vi "Stepper.vi"(8 "error in":errorcluster, 9 "Axis Queue":refnum<queue>, 10 "UI Queue":refnum<queue>) -> (0 "error out":errorcluster)   [LabVIEW 2016, in "SMD-7615.lvlib"]
uses:
  SMD-7615.lvlib
  support/Message Queue/Message Cluster.ctl
  CTL/Stepper Drive Config.ctl
  CTL/SV General.ctl
  CTL/SV Inputs.ctl
  CTL/SV Outputs.ctl
  CTL/Motion IO.ctl
  CTL/Digital Lines (Read).ctl
  CTL/Status.ctl
  CTL/Encoder.ctl
  CTL/Position.ctl
  <vilib>/Motion/PropertyNodes/nimc.createStraightLineMoveInstance.axis.vi
  <vilib>/GPower/Error/Library/Append/AppendSingle.vi
  support/Message Queue/Enqueue Message (Single).vi
  <vilib>/Motion/PropertyNodes/nimc.destroyInterfaceInstance.vi
  <vilib>/ErrorRing/Error Ring.xnode
  support/Message Queue/Message Queue.lvlib
  <resource>/objmgr/nimotion.rc
  <resource>/objmgr/nimcca.rc
  <vilib>/GPower/Error/GPError.lvlib
  LUL-All/LUL-Syslog/LUL-SysLog.lvlib
panel:
  out "Timeout Counter":i32
  out "Stall detected (Software)":bool
  out "Moving ? (Software)":bool
  out "Position":T1
  out "Encoder":T2
  out "Status":T3
  in  "Stop Button":bool
  out "Axis Name":string
  out "Digital Lines (Read)":T4
  out "Motion I/O":T5
  out "dt DAQ Loop (ms)":u32
  out "Axis Config Constant":T6
  out "Last Received SV Update":timestamp
  out "Exit ?":bool
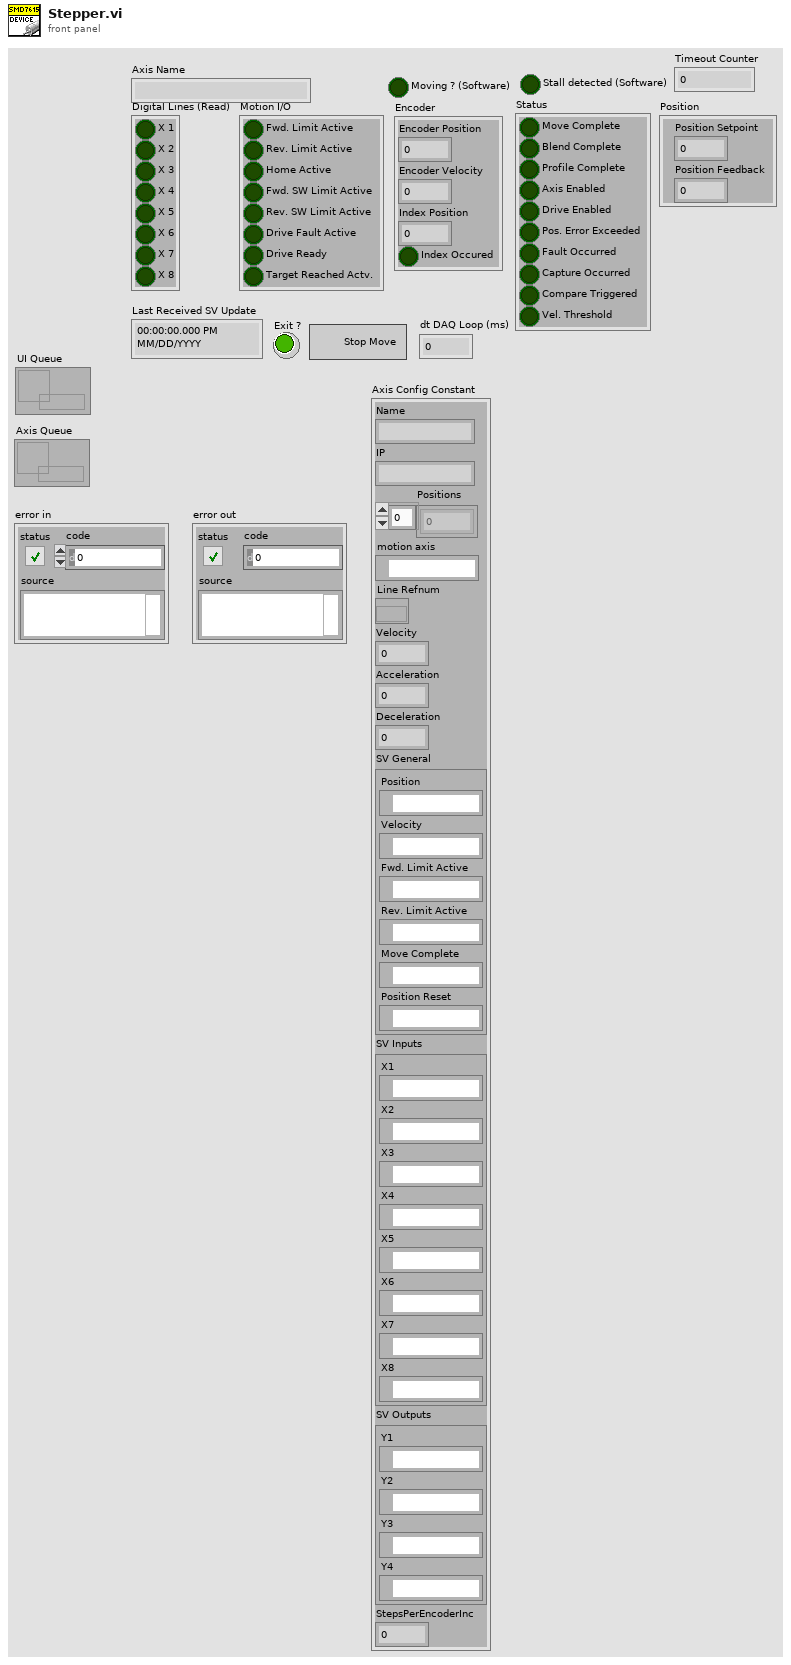
[diagram p1: front panel]
types:
  T1 = typedef "SMD-7615.lvlib/Position.ctl" = cluster{"Position Setpoint":dbl, "Position Feedback":dbl}
  T2 = typedef "SMD-7615.lvlib/Encoder.ctl" = cluster{"Encoder Position":dbl, "Encoder Velocity":dbl, "Index Position":dbl, "Index Occured":bool}
  T3 = typedef "SMD-7615.lvlib/Status.ctl" = cluster{"Move Complete":bool, "Blend Complete":bool, "Profile Complete":bool, "Axis Enabled":bool, "Drive Enabled":bool, "Pos. Error Exceeded":bool, "Fault Occurred":bool, "Capture Occurred":bool, "Compare Triggered":bool, "Vel. Threshold":bool}
  T4 = typedef "SMD-7615.lvlib/Digital Lines (Read).ctl" = cluster{"X 1":bool, "X 2":bool, "X 3":bool, "X 4":bool, "X 5":bool, "X 6":bool, "X 7":bool, "X 8":bool}
  T5 = typedef "SMD-7615.lvlib/Motion IO.ctl" = cluster{"Fwd. Limit Active":bool, "Rev. Limit Active":bool, "Home Active":bool, "Fwd. SW Limit Active":bool, "Rev. SW Limit Active":bool, "Drive Fault Active":bool, "Drive Ready":bool, "Target Reached Actv.":bool}
  T6 = typedef "SMD-7615.lvlib/Stepper Drive Config.ctl" = cluster{"Name":string, "IP":string, "Positions":dbl[], "motion axis ":refnum<k21>, "Line Refnum":refnum<k20>, "Velocity":dbl, "Acceleration":dbl, "Deceleration":dbl, "SV General":T7, "SV Inputs":T8, "SV Outputs":T9, "StepsPerEncoderInc":i32}
  T7 = typedef "SMD-7615.lvlib/SV General.ctl" = cluster{"Position":refnum<k21>, "Velocity":refnum<k21>, "Fwd. Limit Active":refnum<k21>, "Rev. Limit Active":refnum<k21>, "Move Complete":refnum<k21>, "Position Reset":refnum<k21>}
  T8 = typedef "SMD-7615.lvlib/SV Inputs.ctl" = cluster{"X1":refnum<k21>, "X2":refnum<k21>, "X3":refnum<k21>, "X4":refnum<k21>, "X5":refnum<k21>, "X6":refnum<k21>, "X7":refnum<k21>, "X8":refnum<k21>}
  T9 = typedef "SMD-7615.lvlib/SV Outputs.ctl" = cluster{"Y1":refnum<k21>, "Y2":refnum<k21>, "Y3":refnum<k21>, "Y4":refnum<k21>}
  T10 = typedef "Semaphore RefNum" = refnum<k1>
  T11 = typedef "SMD-7615.lvlib/Axis Data.ctl" = cluster{"Motion I/O":T5, "Digital Lines (Read)":T4, "Status":T3, "Encoder":T2, "Position":T1, "Moving ? (Software)":bool, "Stall detected (Software)":bool}
  T12 = enum32{"Invalid", "Standard", "Closed", "Hidden", "Minimized", "Maximized"}
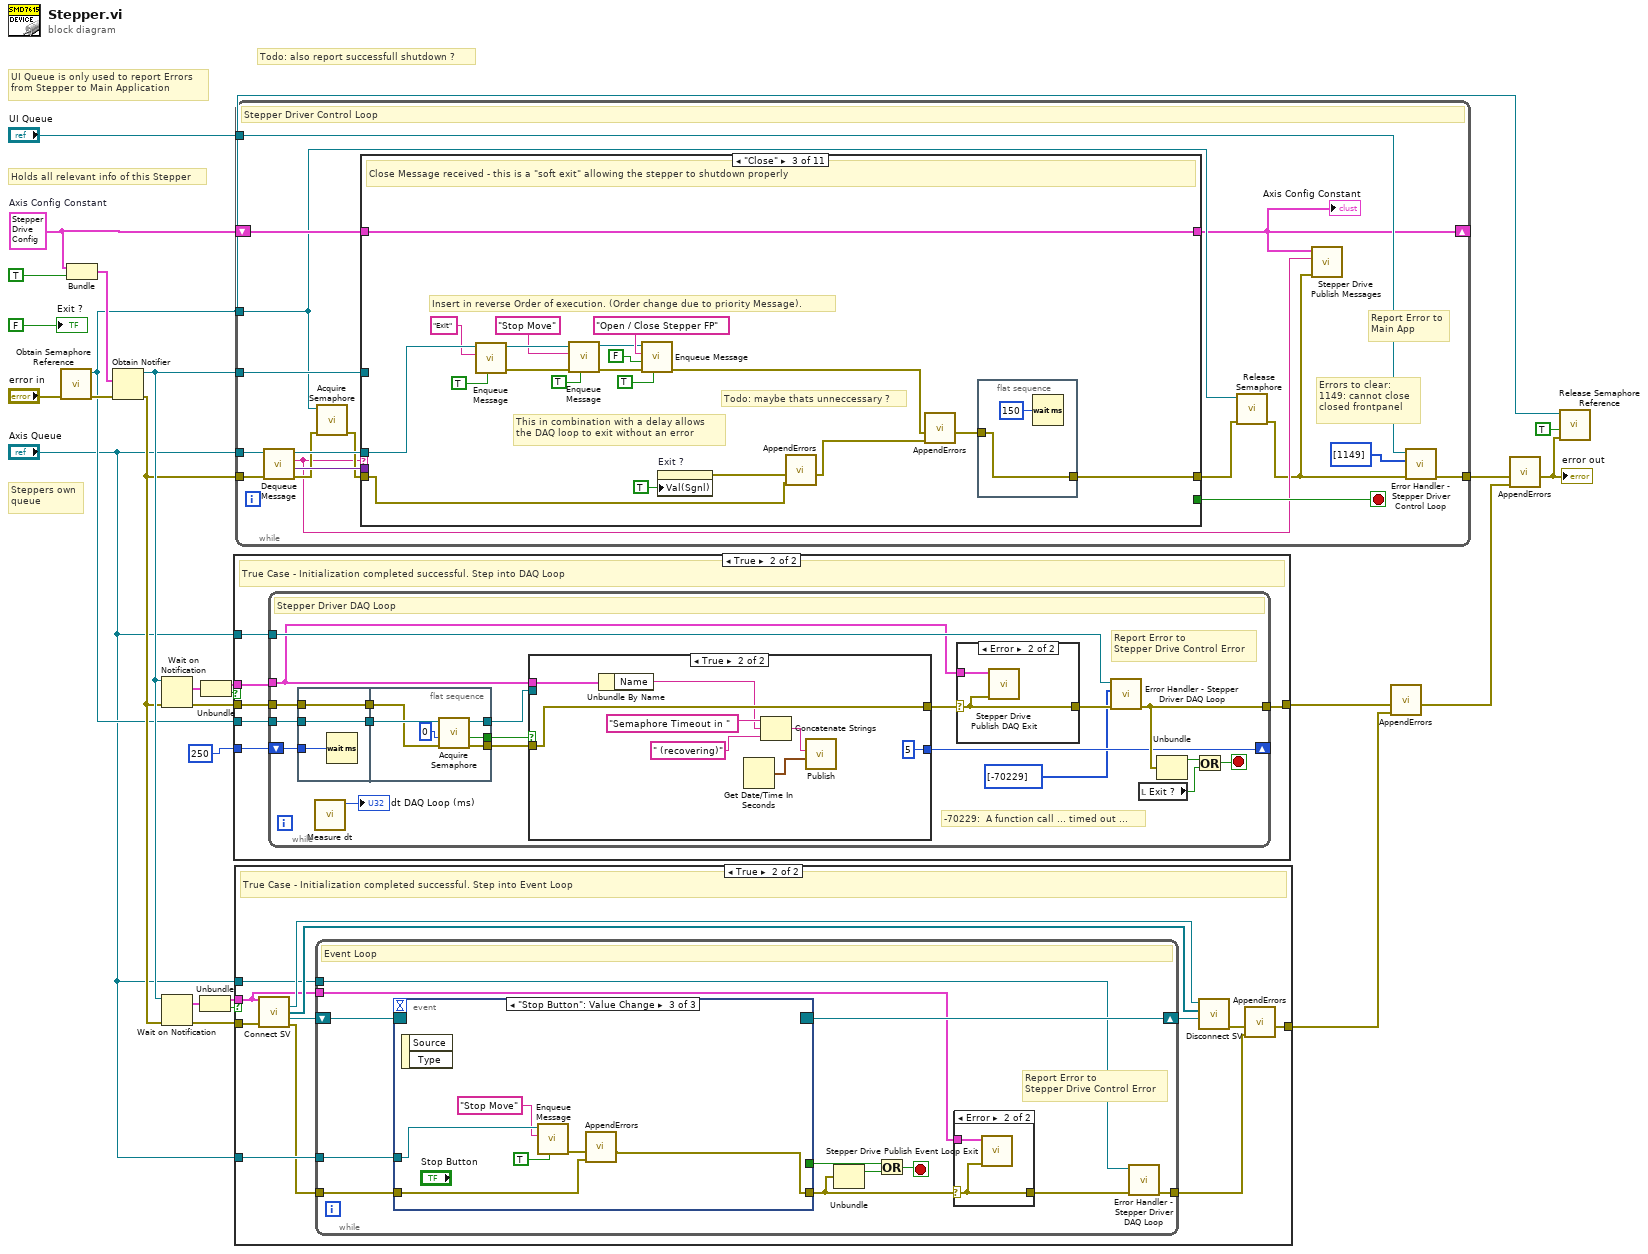
[diagram p0: block diagram]
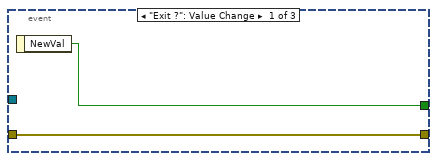
[diagram p4: hidden frame]
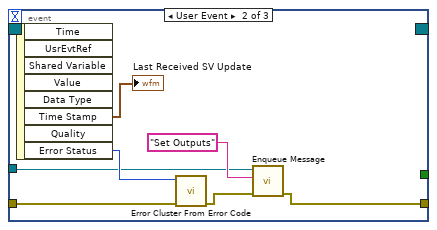
[diagram p5: hidden frame]
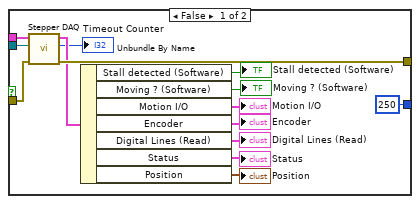
[diagram p8: hidden frame]
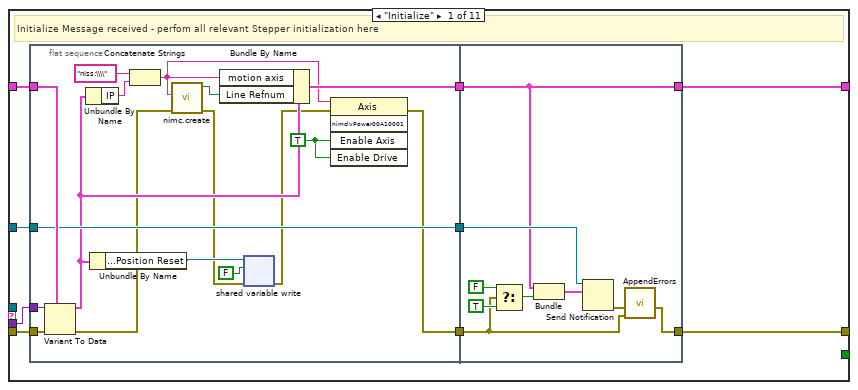
[diagram p9: hidden frame]
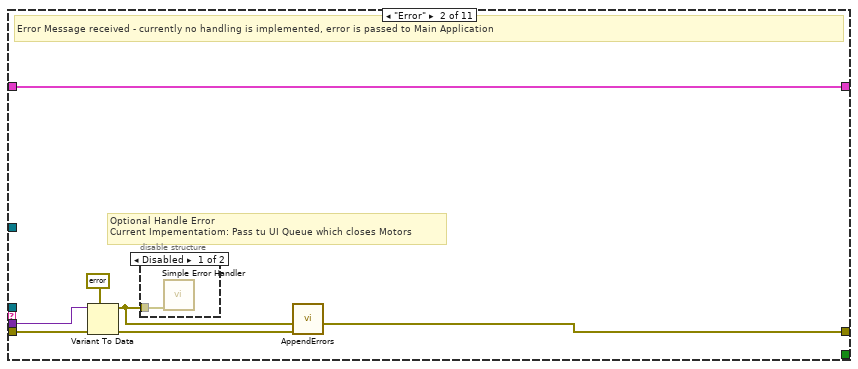
[diagram p10: hidden frame]
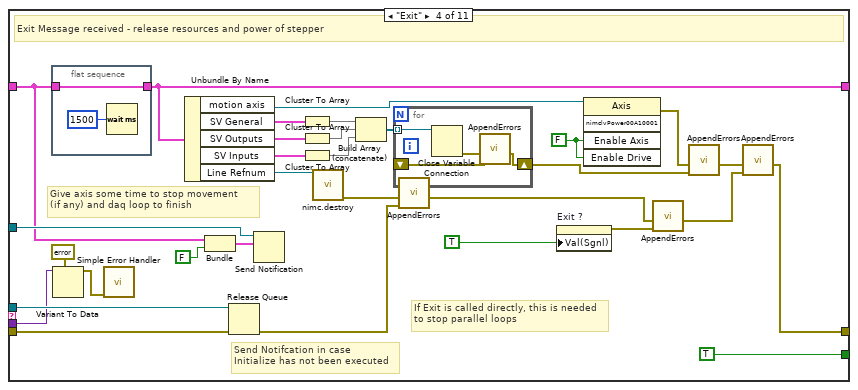
[diagram p12: hidden frame]
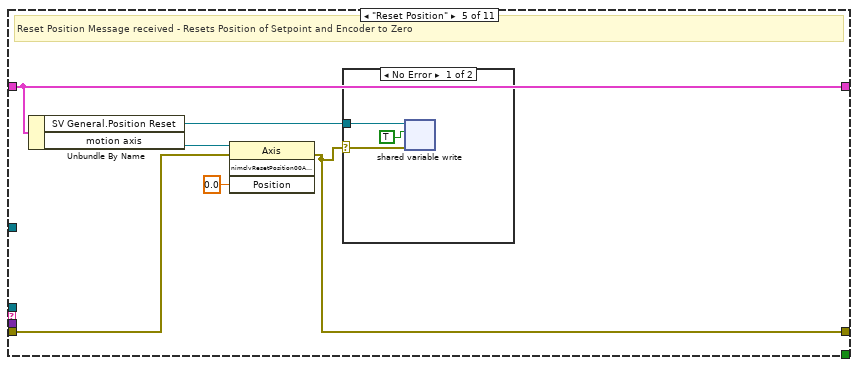
[diagram p13: hidden frame]
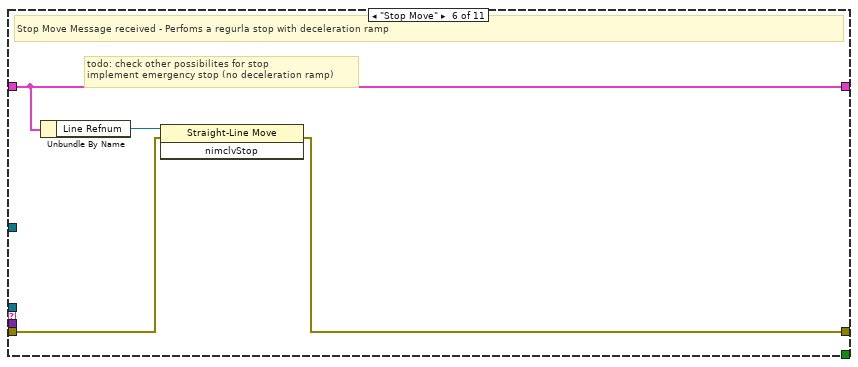
[diagram p15: hidden frame]
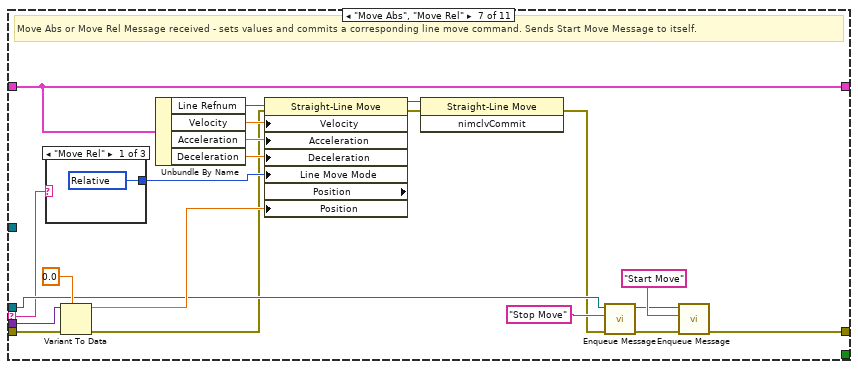
[diagram p16: hidden frame]
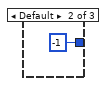
[diagram p17: hidden frame]
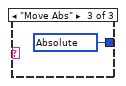
[diagram p18: hidden frame]
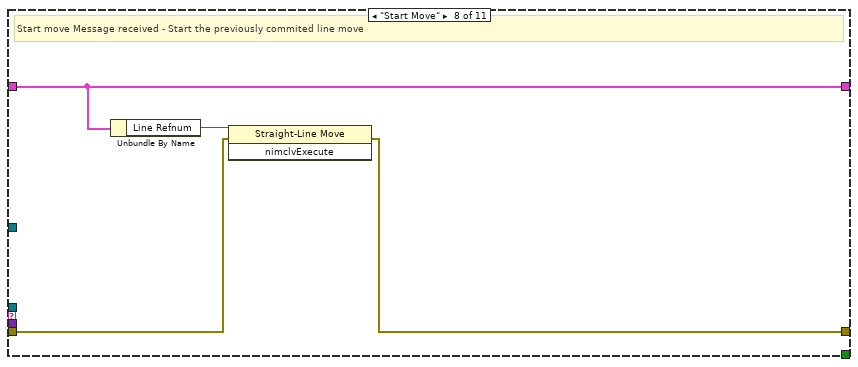
[diagram p19: hidden frame]
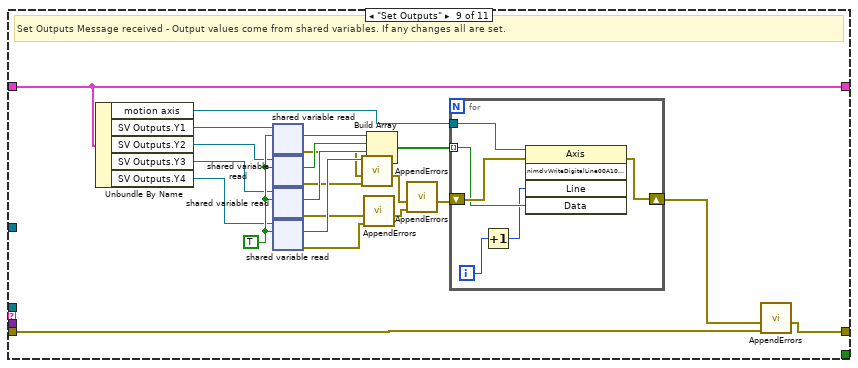
[diagram p20: hidden frame]
diagram:
  w11 = T6 {"Name"="", "IP"="", "Positions"=[], "motion axis "="", "Line Refnum"=refnum, "Velocity"=0.0, "Acceleration"=0.0, "Deceleration"=0.0, "SV General"={"Position"="", "Velocity"="", "Fwd. Limit Active"="", "Rev. Limit Active"="", "Move Complete"="", "Position Reset"=""}, "SV Inputs"={"X1"="", "X2"="", "X3"="", "X4"="", "X5"="", "X6"="", "X7"="", "X8"=""}, "SV Outputs"={"Y1"="", "Y2"="", "Y3"="", "Y4"=""}, "StepsPerEncoderInc"=0}  # Axis Config Constant
  # "Steppers own\nqueue"
  # "Holds all relevant info of this Stepper"
  # "Todo: also report successfull shutdown ?"
  # "UI Queue is only used to report Errors\nfrom Stepper to Main Application"
  n1 = call <vilib>:"Obtain Semaphore Reference.vi"("error in (no error)"="error in") -> ("error out"=w9:errorcluster, "semaphore"=w7:T10)  [unwired: 4 in, 1 out]
  n2 = Bundle("Axis Config Constant"=w11, TRUE) -> (w22:cluster{"Axis Config Constant":T6, bool})  [unwired: 1 in]
  n3 = Obtain Notifier(notification data type=w22, error in (no error)=w9) -> (notifier out=w23:refnum<notifier>, error out=w10:errorcluster)  [unwired: 2 in, 1 out]
  n4 = Wait on Notification(notifier=w23, error in (no error)=w10) -> (notification=w20:cluster{"Axis Config Constant":T6, bool}, error out=w25:errorcluster)  [unwired: 2 in, 2 out]
  n5 = Wait on Notification(notifier=w23, error in (no error)=w10) -> (notification=w17:cluster{"Axis Config Constant":T6, bool}, error out=w24:errorcluster)  [unwired: 2 in, 2 out]
  n6 = Unbundle(w17) -> ("Axis Config Constant"=w15:T6, w16:bool)
  n7 = Unbundle(w20) -> ("Axis Config Constant"=w18:T6, w19:bool)
  n8 = case shown="True" w19 {
    tunnel: [w27 w33] -> w5
    tunnel: "Axis Queue" -> [_ w32]
    tunnel: w25 -> [w27 w31]
    tunnel: w18 -> [_ w30]
    tunnel: w7 -> [_ w29]
    tunnel: u32 250 ("millisecond multiple") -> [_ w28]
    frame False {
      # "False Case - Initialization not successful. Skip DAQ Loop"
    }
    frame True {
      # "True Case - Initialization completed successful. Step into DAQ Loop"
      n9 = while {
        tunnel: w31 -> [w40]
        tunnel: [w51] -> w33
        tunnel: w32 -> [w52]
        tunnel: w30 -> [w35]
        tunnel: w29 -> [w43]
        shift-right: [w38] -> _
        shift-left: w28 -> [w39]
        stop <- w48 stop-if-true
        # "-70229:  A function call ... timed out ..."
        # "Report Error to\nStepper Drive Control Error"
        # "Stepper Driver DAQ Loop"
        n10 = flat-sequence {
          tunnel: w43 -> [w58]
          tunnel: [w58] -> w42
          tunnel: [w57] -> w41
          tunnel: w40 -> [w57]
          tunnel: w39 -> [w56]
          tunnel: [w63] -> w46
          tunnel: [w62] -> w45
          tunnel: [w61] -> w44
          tunnel: w42 -> [w60]
          tunnel: w41 -> [w59]
          frame #0 {
            n11 = Wait (ms)(milliseconds to wait=w56) -> ()  [unwired: 1 out]
          }
          frame #1 {
            n12 = call <vilib>:"Acquire Semaphore.vi"("error in (no error)"=w59, "ms timeout (-1)"=0, "semaphore"=w60) -> ("error out"=w61:errorcluster, "timed out"=w63:bool, "semaphore out"=w62:T10)  [unwired: 2 in]
          }
        }
        n13 = call "Measure dt.vi"() -> ("dt"=→"dt DAQ Loop (ms)":u32)  [unwired: 11 in]
        n14 = case shown="True" w46 {
          tunnel: [w78 w85] -> w37
          tunnel: w35 -> [w68 w83]
          tunnel: w45 -> [w67 _]
          tunnel: w44 -> [w66 w85]
          tunnel: [u32 250 ("millisecond multiple") u32 5 ("millisecond multiple")] -> w38
          frame False {
            n15 = call "Stepper DAQ.vi"("error in"=w66, "semaphore"=w67, "BIBA 2017 Config"=w68) -> ("error out"=w78:errorcluster, "Timeout Counter"=→"Timeout Counter":i32, "Axis Data"=w77:T11)  [unwired: 6 in]
            n16 = Unbundle By Name(w77) -> ("Stall detected (Software)"=→"Stall detected (Software)":bool, "Moving ? (Software)"=→"Moving ? (Software)":bool, "Motion I/O"=→"Motion I/O":T5, "Encoder"=→"Encoder":T2, "Digital Lines (Read)"=→"Digital Lines (Read)":T4, "Status"=→"Status":T3, "Position"=→"Position":T1)
          }
          frame True {
            n17 = Unbundle By Name(w83) -> ("Name"=w81:string)
            n18 = Get Date/Time In Seconds() -> (seconds since 1Jan1904=w84:timestamp)
            n19 = Concatenate Strings("Semaphore Timeout in " ("Message"), w81, " (recovering)" ("string")) -> (w80:string)
            n20 = call "Publish.vi"("current time"=w84, "Message"=w80) -> ()  [unwired: 9 in, 1 out]
          }
        }
        n21 = case shown="Error" w37 {
          selector: w37 -> [w53 w55]
          tunnel: [w53 w55] -> w36
          tunnel: w35 -> [_ w54]
          frame No Error {
          }
          frame Error {
            n22 = call "Stepper Drive Publish DAQ Exit.vi"("error in (no error)"=w55, "Axis Config Constant"=w54) -> ()  [unwired: 10 in]
          }
        }
        n23 = call "Error Handler - Stepper Driver DAQ Loop.vi"("error in (no error)"=w36, "Ignore Errors (Runtime)"=i32[] [-70229], "Message Queue"=w52) -> ("dup error in"=w51:errorcluster)  [unwired: 7 in, 1 out]
        n24 = local read "Exit ?"() -> (w49:bool)
        n25 = Unbundle(w51) -> ("status"=w50:bool)  [unwired: 2 out]
        n26 = Or(x=w50, y=w49) -> (x .or. y?=w48:bool)
      }
    }
  }
  n27 = case shown="True" w16 {
    tunnel: "Axis Queue" -> [_ w99]
    tunnel: [w87 w91] -> w4
    tunnel: w24 -> [w87 w98]
    tunnel: w15 -> [_ w88]
    tunnel: "Axis Queue" -> [_ w89]
    frame False {
      # "False Case - Initialization not successful. Skip Event Loop"
    }
    frame True {
      # "True Case - Initialization completed successful. Step into Event Loop"
      n28 = call "Connect SV.vi"("Axis Config in"=w88, "Error In"=w98) -> ("shared variable value change notification"=w95:refnum<user-event>, "Shared Variables"=w93:refnum<k21>[], "Event Registration Refnum"=w96:refnum<event-registration>, "Error Out"=w97:errorcluster)  [unwired: 9 in, 1 out]
      n29 = while {
        tunnel: w99 -> [w109]
        tunnel: w97 -> [w111]
        tunnel: [w104] -> w92
        shift-right: [w108] -> w94
        shift-left: w96 -> [w110]
        tunnel: w89 -> [w102]
        tunnel: w88 -> [w101]
        stop <- w106 stop-if-true
        # "Report Error to\nStepper Drive Control Error"
        # "Event Loop"
        n30 = event shown="[2] \"Stop Button\": Value Change" {
          selector: w110 -> [_ _ _]
          dyn-events: [_ _ _] -> w108
          timeout: _ -> [_ _ _]
          tunnel: w111 -> [w116 w121 w125]
          tunnel: [w116 w117 w126] -> w103
          tunnel: w109 -> [_ w119 w128]
          tunnel: [w115 _ _] -> w105
          event "Exit ?": Value Change {
            n31 = event-data() -> ("NewVal"=w115:bool)  [unwired: 1 in]
          }
          event User Event {
            n32 = event-data() -> ("Time Stamp"=→"Last Received SV Update":timestamp, "Error Status"=w120:i32)  [unwired: 1 in, 6 out]
            n33 = call <vilib>:"Error Cluster From Error Code.vi"("error in (no error)"=w121, "error code (0)"=w120) -> ("error out"=w122:errorcluster)  [unwired: 1 in, 6 out]
            n34 = call-poly "Enqueue Message.vi"("error in (no error)"=w122, "Message"="Set Outputs", "Message Queue"=w119) -> ("error out"=w117:errorcluster)  [unwired: 7 in, 1 out]
          }
          event "Stop Button": Value Change {
            n35 = event-data() -> ()  [unwired: 1 in, 2 out]
            n36 = call-poly "Enqueue Message.vi"("Priority Message? (F)"=TRUE, "Message"="Stop Move", "Message Queue"=w128) -> ("error out"=w124:errorcluster)  [unwired: 7 in, 1 out]
            n37 = call-poly <vilib>:"AppendErrors.vi"("Error to append"=w125, "Error in"=w124) -> ("Appended errors out"=w126:errorcluster)  [unwired: 9 in]
          }
        }
        n38 = Unbundle(w103) -> ("status"=w107:bool)  [unwired: 2 out]
        n39 = Or(x=w105, y=w107) -> (x .or. y?=w106:bool)
        n40 = case shown="Error" w103 {
          selector: w103 -> [w112 w113]
          tunnel: w101 -> [_ w114]
          tunnel: [w112 w113] -> w100
          frame No Error {
          }
          frame Error {
            n41 = call "Stepper Drive Publish Event Loop Exit.vi"("error in (no error)"=w113, "Axis Config Constant"=w114) -> ()  [unwired: 10 in]
          }
        }
        n42 = call "Error Handler - Stepper Driver DAQ Loop.vi"("error in (no error)"=w100, "Message Queue"=w102) -> ("dup error in"=w104:errorcluster)  [unwired: 8 in, 1 out]
      }
      n43 = call "Disconnect SV.vi"("Event Registration Refnum"=w94, "Shared Variables"=w93, "User Event in"=w95) -> ("error out"=w90:errorcluster)  [unwired: 8 in]
      n44 = call-poly <vilib>:"AppendErrors.vi"("Error to append"=w92, "Error in"=w90) -> ("Appended errors out"=w91:errorcluster)  [unwired: 9 in]
    }
  }
  n45 = while {
    tunnel: "Axis Queue" -> [w146]
    tunnel: w10 -> [w145]
    tunnel: [w141] -> w13
    shift-right: [w132] -> _
    shift-left: w11 -> [w142]
    tunnel: "UI Queue" -> [w140]
    tunnel: w23 -> [w138]
    tunnel: w7 -> [w133]
    stop <- w143 stop-if-true
    # "Report Error to\nMain App"
    # "Errors to clear:\n1149: cannot close \nclosed frontpanel"
    # "Stepper Driver Control Loop"
    n46 = call "Dequeue Message.vi"("error in (no error)"=w145, "Message Queue"=w146) -> ("error out"=w136:errorcluster, "Message Data"=w144:variant, "Message"=w131:string, "dup Message Queue"=w139:refnum<queue>)  [unwired: 6 in]
    n47 = call <vilib>:"Acquire Semaphore.vi"("error in (no error)"=w136, "semaphore"=w133) -> ("error out"=w135:errorcluster)  [unwired: 3 in, 2 out]
    n48 = case shown="\"Close\"" w131 {
      selector: w131 -> [_ _ _ _ _ _ w266 _ _ _ w339]
      tunnel: w144 -> [w154 w186 _ w238 _ _ w279 _ _ w326 _]
      tunnel: w135 -> [w155 w185 w194 w240 w251 w261 w282 w287 w297 w327 w335]
      tunnel: [w153 w184 w200 w217 w250 w258 w262 w286 w299 w318 w334] -> w134
      tunnel: w139 -> [_ _ w208 w239 _ _ w269 _ _ _ _]
      tunnel: [_ _ _ TRUE _ _ _ _ _ _ _] -> w143
      tunnel: w142 -> [w152 w188 w209 w213 w253 w260 w281 w289 w311 w321 w338]
      tunnel: [w150 w188 w209 w216 w253 w260 w281 w289 w311 w321 w338] -> w132
      tunnel: w138 -> [w147 _ _ w214 _ _ _ _ _ _ _]
      frame "Initialize" {
        # "Initialize Message received - perfom all relevant Stepper initialization here"
        n49 = flat-sequence {
          tunnel: w155 -> [w172]
          tunnel: w154 -> [w171]
          tunnel: w152 -> [w168]
          tunnel: [w163] -> w151
          tunnel: [w165] -> w149
          tunnel: [w166] -> w148
          tunnel: w147 -> [w166]
          tunnel: [w173] -> w153
          tunnel: w151 -> [w174]
          tunnel: [w178] -> w150
          tunnel: w149 -> [w178]
          tunnel: w148 -> [w179]
          frame #0 {
            w162 = TRUE ("Enable Axis")
            n50 = Variant To Data(error in=w172, type=w168, Variant=w171) -> (data=w160:T6, error out=w156:errorcluster)
            n51 = Unbundle By Name(w160) -> ("IP"=w169:string)
            n52 = Unbundle By Name(w160) -> ("SV General.Position Reset"=w159:refnum<k21>)
            n53 = Concatenate Strings("niss:\\\\" ("string"), w169) -> (w164:string)
            n54 = call-poly <vilib>:"nimc.create.vi"("error in"=w156, "axis"=w164) -> ("error out"=w158:errorcluster, "line"=w167:refnum<k20>)  [unwired: 7 in, 1 out]
            n55 = Bundle By Name(cluster=w160, "motion axis"=w164, "Line Refnum"=w167) -> (w165:T6)
            n56 = shared-variable-write(w159, w158, FALSE) -> (w157:errorcluster)  [unwired: 1 out]
            n57 = invoke class="Axis" method="nimclvPower00A10001"(reference=w164, error in=w157, "Enable Axis"=w162, "Enable Drive"=w162) -> (error out=w163:errorcluster)  [unwired: 1 in, 4 out]
          }
          frame #1 {
            n58 = Select(t=FALSE ("Stepper Init Done"), s=w174, f=TRUE) -> (s? t:f=w177:bool)
            n59 = Bundle("Axis Config Constant"=w178, "f"=w177) -> (w176:cluster{"Axis Config Constant":T6, "f":bool})  [unwired: 1 in]
            n60 = Send Notification(notification=w176, notifier=w179) -> (error out=w175:errorcluster)  [unwired: 1 in, 1 out]
            n61 = call-poly <vilib>:"AppendErrors.vi"("Error to append"=w174, "Error in"=w175) -> ("Appended errors out"=w173:errorcluster)  [unwired: 9 in]
          }
        }
      }
      frame "Error" {
        # "Optional Handle Error\nCurrent Impementatiom: Pass tu UI Queue which closes Motors"
        # "Error Message received - currently no handling is implemented, error is passed to Main Application"
        n62 = Variant To Data(error in=w185, type=errorcluster {"status"=FALSE, "code"=0, "source"=""} ("error constant"), Variant=w186) -> (data=w183:errorcluster, error out=w182:errorcluster)
        n63 = disable-structure shown="Disabled" {
          disable-tunnel: w183 -> [w189 _]
          frame Disabled {
            n64 = call <vilib>:"Simple Error Handler.vi"("error in (no error)"=w189) -> ()  [unwired: 4 in, 5 out]
          }
          frame Enabled {
          }
        }
        n65 = call-poly <vilib>:"AppendErrors.vi"("Error to append"=w182, "Error in"=w183) -> ("Appended errors out"=w184:errorcluster)  [unwired: 9 in]
      }
      frame "Close" {
        # "Todo: maybe thats unneccessary ?"
        # "This in combination with a delay allows\nthe DAQ loop to exit without an error"
        # "Insert in reverse Order of execution. (Order change due to priority Message)."
        # "Close Message received - this is a \"soft exit\" allowing the stepper to shutdown properly"
        n66 = call-poly "Enqueue Message.vi"("Priority Message? (F)"=TRUE, "Message"="Exit", "Message Queue"=w208) -> ("error out"=w203:errorcluster, "dup Message Queue"=w204:refnum<queue>)  [unwired: 7 in]
        n67 = call-poly "Enqueue Message.vi"("Priority Message? (F)"=TRUE, "error in (no error)"=w203, "Message"="Stop Move", "Message Queue"=w204) -> ("error out"=w197:errorcluster, "dup Message Queue"=w198:refnum<queue>)  [unwired: 6 in]
        n68 = call-poly "Enqueue Message.vi"("Priority Message? (F)"=TRUE, "error in (no error)"=w197, "Message Data"=FALSE, "Message"="Open / Close Stepper FP", "Message Queue"=w198) -> ("error out"=w192:errorcluster)  [unwired: 5 in, 1 out]
        n69 = property on="Exit ?" class="Bool (strict)"("Val(Sgnl)"=TRUE ("Value (Signaling)")) -> (error out=w195:errorcluster)  [unwired: 2 in, 1 out]
        n70 = call-poly <vilib>:"AppendErrors.vi"("Error to append"=w194, "Error in"=w195) -> ("Appended errors out"=w191:errorcluster)  [unwired: 9 in]
        n71 = call-poly <vilib>:"AppendErrors.vi"("Error to append"=w191, "Error in"=w192) -> ("Appended errors out"=w193:errorcluster)  [unwired: 9 in]
        n72 = flat-sequence {
          tunnel: [w210] -> w200
          tunnel: w193 -> [w210]
          frame #0 {
            n73 = Wait (ms)(milliseconds to wait=u32 150) -> ()  [unwired: 1 out]
          }
        }
      }
      frame "Exit" {
        w228 = FALSE ("Enable Axis")
        # "Send Notifcation in case\nInitialize has not been executed"
        # "Give axis some time to stop movement \n(if any) and daq loop to finish"
        # "If Exit is called directly, this is needed\nto stop parallel loops"
        # "Exit Message received - release resources and power of stepper"
        n74 = flat-sequence {
          tunnel: w213 -> [w243]
          tunnel: [w243] -> w216
          frame #0 {
            n75 = Wait (ms)(milliseconds to wait=u32 1500) -> ()  [unwired: 1 out]
          }
        }
        n76 = Variant To Data(type=errorcluster {"status"=FALSE, "code"=0, "source"=""} ("error constant"), Variant=w238) -> (data=w241:errorcluster)  [unwired: 1 in, 1 out]
        n77 = call <vilib>:"Simple Error Handler.vi"("error in (no error)"=w241) -> ()  [unwired: 4 in, 5 out]
        n78 = Unbundle By Name(w216) -> ("motion axis"=w227:refnum<k21>, "SV General"=w236:T7, "SV Outputs"=w232:T9, "SV Inputs"=w233:T8, "Line Refnum"=w237:refnum<k20>)
        n79 = Bundle("Axis Config Constant"=w213, FALSE) -> (w215:cluster{"Axis Config Constant":T6, bool})  [unwired: 1 in]
        n80 = Release Queue(queue=w239, error in (no error)=w240) -> (error out=w222:errorcluster)  [unwired: 1 in, 2 out]
        n81 = Send Notification(notification=w215, notifier=w214) -> ()  [unwired: 1 in, 2 out]
        n82 = Cluster To Array(cluster=w236) -> (array=w235:refnum<k21>[])
        n83 = Cluster To Array(cluster=w232) -> (array=w231:refnum<k21>[])
        n84 = Cluster To Array(cluster=w233) -> (array=w230:refnum<k21>[])
        n85 = call-poly <vilib>:"nimc.destroy.vi"("motion handle"=w237) -> ("error out"=w223:errorcluster)  [unwired: 10 in]
        n86 = Build Array (concatenate)(w235, w231, w230) -> (w234:refnum<k21>[])
        n87 = for {
          tunnel: w234 -> [w248] mode=indexing
          shift-right: [w246] -> w224
          shift-left: _ -> [w245]
          n88 = Close Variable Connection(11:w248) -> (0:w247:errorcluster)  [unwired: 1 in]
          n89 = call-poly <vilib>:"AppendErrors.vi"("Error to append"=w245, "Error in"=w247) -> ("Appended errors out"=w246:errorcluster)  [unwired: 9 in]
        }
        n90 = call-poly <vilib>:"AppendErrors.vi"("Error to append"=w222, "Error in"=w223) -> ("Appended errors out"=w220:errorcluster)  [unwired: 9 in]
        n91 = property on="Exit ?" class="Bool (strict)"("Val(Sgnl)"=TRUE ("Value (Signaling)")) -> (error out=w221:errorcluster)  [unwired: 2 in, 1 out]
        n92 = invoke class="Axis" method="nimclvPower00A10001"(reference=w227, "Enable Axis"=w228, "Enable Drive"=w228) -> (error out=w225:errorcluster)  [unwired: 2 in, 4 out]
        n93 = call-poly <vilib>:"AppendErrors.vi"("Error to append"=w221, "Error in"=w220) -> ("Appended errors out"=w219:errorcluster)  [unwired: 9 in]
        n94 = call-poly <vilib>:"AppendErrors.vi"("Error to append"=w224, "Error in"=w225) -> ("Appended errors out"=w218:errorcluster)  [unwired: 9 in]
        n95 = call-poly <vilib>:"AppendErrors.vi"("Error to append"=w219, "Error in"=w218) -> ("Appended errors out"=w217:errorcluster)  [unwired: 9 in]
      }
      frame "Reset Position" {
        # "Reset Position Message received - Resets Position of Setpoint and Encoder to Zero"
        n96 = Unbundle By Name(w253) -> ("SV General.Position Reset"=w249:refnum<k21>, "motion axis"=w252:refnum<k21>)
        n97 = invoke class="Axis" method="nimclvResetPosition00A10001"(reference=w252, error in=w251, "Position"=0.0) -> (error out=w250:errorcluster)  [unwired: 1 in, 3 out]
        n98 = case shown="No Error" w250 {
          selector: w250 -> [w256 _]
          tunnel: w249 -> [w257 _]
          frame No Error {
            n99 = shared-variable-write(w257, w256, TRUE) -> ()  [unwired: 2 out]
          }
          frame Error {
          }
        }
      }
      frame "Stop Move" {
        # "todo: check other possibilites for stop\nimplement emergency stop (no deceleration ramp)"
        # "Stop Move Message received - Perfoms a regurla stop with deceleration ramp"
        n100 = Unbundle By Name(w260) -> ("Line Refnum"=w259:refnum<k20>)
        n101 = invoke class="Straight-Line Move" method="nimclvStop"(reference=w259, error in=w261) -> (error out=w258:errorcluster)  [unwired: 1 in, 2 out]
      }
      frame "Move Abs", "Move Rel" {
        # "Move Abs or Move Rel Message received - sets values and commits a corresponding line move command. Sends Start Move Message to itself."
        n102 = case shown="\"Move Rel\"" w266 {
          tunnel: [w283 -1 ("Move Mode") w285] -> w272
          frame "Move Rel" {
            w283 = 10551344 items=["Absolute"=10551337, "Relative"=10551344, "Relative To Capture"=10551345, "Velocity"=10551346] ("Move Mode")
          }
          frame Default {
          }
          frame "Move Abs" {
            w285 = 10551337 items=["Absolute"=10551337, "Relative"=10551344, "Relative To Capture"=10551345, "Velocity"=10551346] ("Move Mode")
          }
        }
        n103 = Variant To Data(error in=w282, type=0.0 ("Position"), Variant=w279) -> (data=w271:dbl, error out=w268:errorcluster)
        n104 = Unbundle By Name(w281) -> ("Line Refnum"=w276:refnum<k20>, "Velocity"=w275:dbl, "Acceleration"=w274:dbl, "Deceleration"=w273:dbl)
        n105 = property class="Straight-Line Move" props=["Velocity", "Acceleration", "Deceleration", "Line Move Mode", "Position", "Position"](reference=w276, error in=w268, "Velocity"=w275, "Acceleration"=w274, "Deceleration"=w273, "Line Move Mode"=w272, "Position"=w271) -> (reference out=w278:refnum<k20>, error out=w277:errorcluster)  [unwired: 1 out]
        n106 = invoke class="Straight-Line Move" method="nimclvCommit"(reference=w278, error in=w277) -> (error out=w267:errorcluster)  [unwired: 1 in, 2 out]
        n107 = call-poly "Enqueue Message.vi"("error in (no error)"=w267, "Message"="Stop Move", "Message Queue"=w269) -> ("error out"=w263:errorcluster, "dup Message Queue"=w264:refnum<queue>)  [unwired: 7 in]
        n108 = call-poly "Enqueue Message.vi"("error in (no error)"=w263, "Message"="Start Move", "Message Queue"=w264) -> ("error out"=w262:errorcluster)  [unwired: 7 in, 1 out]
      }
      frame "Start Move" {
        # "Start move Message received - Start the previously commited line move"
        n109 = Unbundle By Name(w289) -> ("Line Refnum"=w288:refnum<k20>)
        n110 = invoke class="Straight-Line Move" method="nimclvExecute"(reference=w288, error in=w287) -> (error out=w286:errorcluster)  [unwired: 1 in, 2 out]
      }
      frame "Set Outputs" {
        w310 = TRUE
        # "Set Outputs Message received - Output values come from shared variables. If any changes all are set."
        n111 = Unbundle By Name(w311) -> ("motion axis"=w300:refnum<k21>, "SV Outputs.Y1"=w309:refnum<k21>, "SV Outputs.Y2"=w308:refnum<k21>, "SV Outputs.Y3"=w307:refnum<k21>, "SV Outputs.Y4"=w306:refnum<k21>)
        n112 = shared-variable-read(w309, w310) -> (w296:errorcluster, w305:bool)  [unwired: 1 in, 2 out]
        n113 = shared-variable-read(w308, w310) -> (w295:errorcluster, w304:bool)  [unwired: 1 in, 2 out]
        n114 = shared-variable-read(w307, w310) -> (w294:errorcluster, w303:bool)  [unwired: 1 in, 2 out]
        n115 = shared-variable-read(w306, w310) -> (w293:errorcluster, w302:bool)  [unwired: 1 in, 2 out]
        n116 = call-poly <vilib>:"AppendErrors.vi"("Error to append"=w295, "Error in"=w296) -> ("Appended errors out"=w292:errorcluster)  [unwired: 9 in]
        n117 = call-poly <vilib>:"AppendErrors.vi"("Error to append"=w293, "Error in"=w294) -> ("Appended errors out"=w290:errorcluster)  [unwired: 9 in]
        n118 = Build Array(w305, w304, w303, w302) -> (w301:bool[])
        n119 = call-poly <vilib>:"AppendErrors.vi"("Error to append"=w290, "Error in"=w292) -> ("Appended errors out"=w291:errorcluster)  [unwired: 9 in]
        n120 = for {
          tunnel: w301 -> [w316] mode=indexing
          tunnel: w300 -> [w315]
          shift-right: [w312] -> w298
          shift-left: w291 -> [w317]
          i -> [w314]
          n121 = Increment(x=w314) -> (x+1=w313:i32)
          n122 = invoke class="Axis" method="nimclvWriteDigitalLine00A10001"(reference=w315, error in=w317, "Line"=w313, "Data"=w316) -> (error out=w312:errorcluster)  [unwired: 1 in, 4 out]
        }
        n123 = call-poly <vilib>:"AppendErrors.vi"("Error to append"=w297, "Error in"=w298) -> ("Appended errors out"=w299:errorcluster)  [unwired: 9 in]
      }
      frame "Open / Close Stepper FP" {
        # "Open / Close Stepper FP Message received - Opens or closes VI Frontpanel. This is intended to be a debugging feature"
        n124 = Unbundle By Name(w321) -> ("Name"=→"Axis Name":string)
        n125 = control-ref of="This VI"() -> (w323:refnum<vi>)
        n126 = Variant To Data(error in=w327, type=TRUE, Variant=w326) -> (data=w324:bool, error out=w319:errorcluster)
        n127 = case shown="True" w324 {
          tunnel: w323 -> [w329 w331]
          tunnel: [w328 w330] -> w320
          frame False {
            n128 = invoke class="VI" method="FP.Close"(reference=w329) -> (error out=w328:errorcluster)  [unwired: 2 in, 2 out]
          }
          frame True {
            n129 = invoke class="VI" method="FP.Open"(reference=w331, "Activate"=TRUE ("Activate?"), "State"=T12."Standard") -> (error out=w330:errorcluster)  [unwired: 2 in, 4 out]
          }
        }
        n130 = call-poly <vilib>:"AppendErrors.vi"("Error to append"=w319, "Error in"=w320) -> ("Appended errors out"=w318:errorcluster)  [unwired: 9 in]
      }
      frame Default {
        # "Anything else received - This is invalid and handled as an Error"
        n131 = Unbundle By Name(w338) -> ("Name"=w337:string)
        n132 = xnode "Error Ring"("parameter 0"=w339, "parameter 1"=w337) -> ("error out"=w336:errorcluster)
        n133 = call-poly <vilib>:"AppendErrors.vi"("Error to append"=w335, "Error in"=w336) -> ("Appended errors out"=w334:errorcluster)  [unwired: 9 in]
      }
    }
    "Axis Config Constant" <- w132
    n134 = call <vilib>:"Release Semaphore.vi"("error in (no error)"=w134, "semaphore"=w133) -> ("error out"=w130:errorcluster)  [unwired: 4 in, 1 out]
    n135 = call "Stepper Drive Publish Messages.vi"("error in (no error)"=w130, "Message"=w131, "Axis Config Constant"=w132) -> ()  [unwired: 9 in]
    n136 = call "Error Handler - Stepper Driver Control Loop.vi"("error in (no error)"=w130, "Ignore Errors (Runtime)"=i32[] [1149], "Message Queue"=w140) -> ("dup error in"=w141:errorcluster)  [unwired: 7 in, 1 out]
  }
  n137 = call-poly <vilib>:"AppendErrors.vi"("Error to append"=w4, "Error in"=w5) -> ("Appended errors out"=w12:errorcluster)  [unwired: 9 in]
  n138 = call-poly <vilib>:"AppendErrors.vi"("Error to append"=w12, "Error in"=w13) -> ("Appended errors out"=w3:errorcluster)  [unwired: 9 in]
  "error out" <- w3
  n139 = call <vilib>:"Release Semaphore Reference.vi"("error in (no error)"=w3, "force destroy? (F)"=TRUE, "semaphore"=w7) -> ()  [unwired: 7 in, 2 out]
  "Exit ?" <- FALSE ("Exit ?")
